vi "Handle.vi"(10 "log record":T1 {"timestamp" format="%<%x %.3X>T"}, 11 "logger in":refnum<class "Logger.lvclass">) -> (3 "logger out":refnum<class "Logger.lvclass">)   [LabVIEW 2024, in "Logging.lvlib" / "Logger.lvclass"]
uses:
  Logger.lvclass
  Log Record.ctl
  Internal Log Levels.ctl
  Logger.lvclass/Logger.ctl
  Failure Popup.vi
  <vilib>/ErrorRing/Error Ring.xnode
  Handlers/Handler/Handler.lvclass
  Logging.lvlib
panel:
  # "Connector Pane"
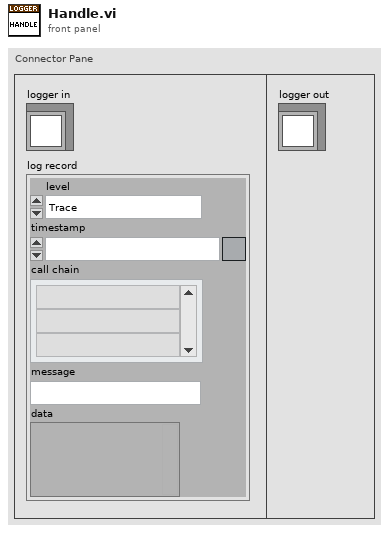
[diagram p1: front panel]
types:
  T1 = typedef "Logging.lvlib/Log Record.ctl" = cluster{"level":T2, "timestamp":timestamp, "call chain":string[], "message":string, "data":variant}
  T2 = typedef "Logging.lvlib/Internal Log Levels.ctl" = enum16{"Trace", "Debug", "Info", "Warning", "Error", "Critical", "Internal"}
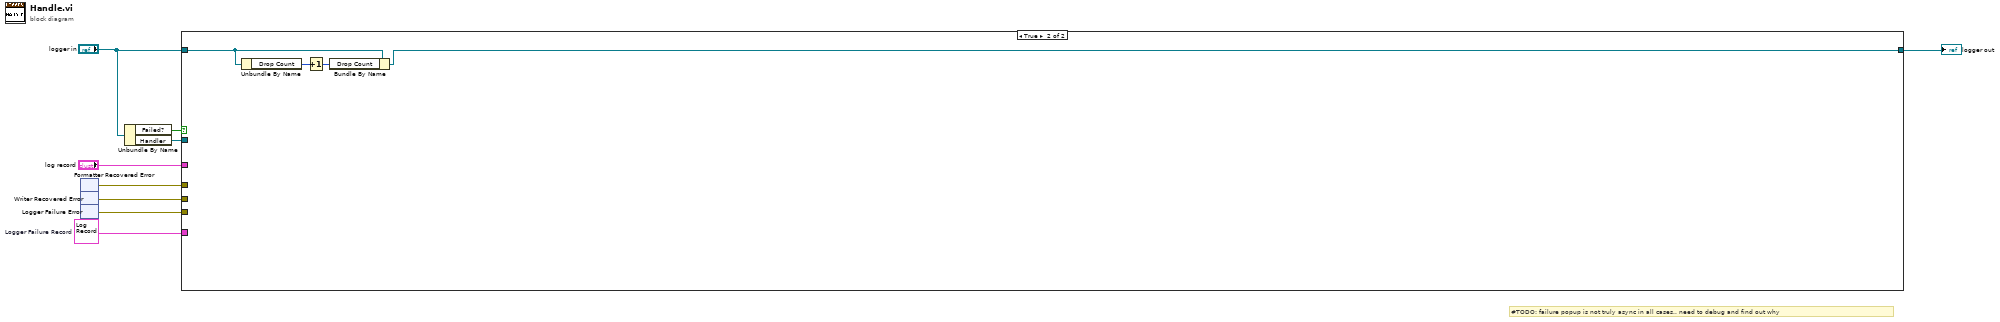
[diagram p0: block diagram]
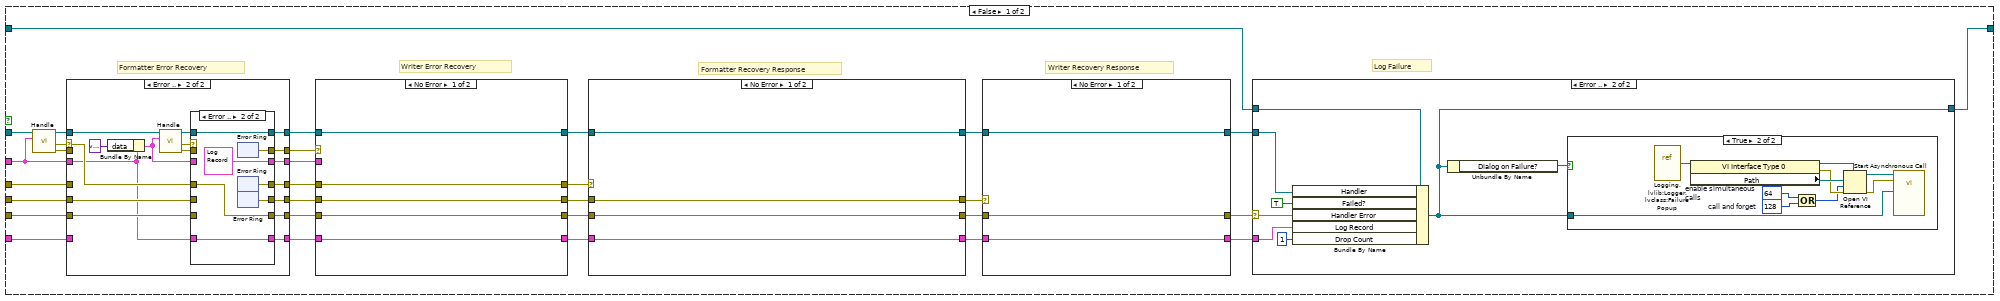
[diagram p2: hidden frame]
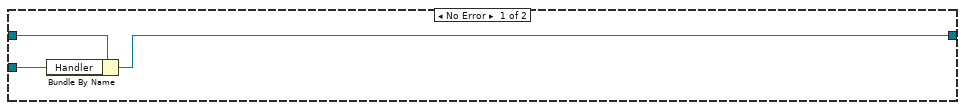
[diagram p3: hidden frame]
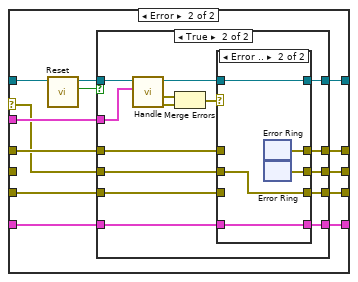
[diagram p7: hidden frame]
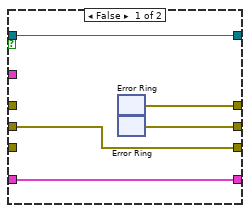
[diagram p8: hidden frame]
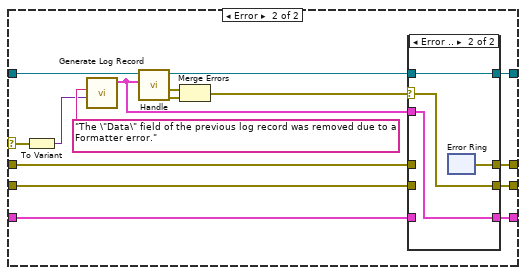
[diagram p10: hidden frame]
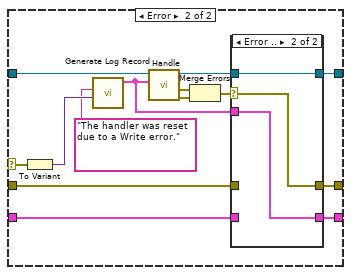
[diagram p12: hidden frame]
diagram:
  w9 = T1 {"level"=enum."Trace", "timestamp"=timestamp(0 s since 1904-01-01), "call chain"=[], "message"="", "data"=variant}  # Logger Failure Record
  # "#TODO: failure popup is not truly async in all cases.. need to debug and find out why"
  n1 = xnode "Formatter Recovered Error"() -> ("error out"=w6:errorcluster)
  n2 = xnode "Writer Recovered Error"() -> ("error out"=w7:errorcluster)
  n3 = xnode "Logger Failure Error"() -> ("error out"=w8:errorcluster)
  n4 = Unbundle By Name("logger in") -> ("Failed?"=w1:bool, "Handler"=w5:refnum<class "Handler.lvclass">)
  n5 = case shown="True" w1 {
    tunnel: w9 -> [w38 _]
    tunnel: w8 -> [w33 _]
    tunnel: w7 -> [w32 _]
    tunnel: w6 -> [w30 _]
    tunnel: w5 -> [w15 _]
    tunnel: "log record" -> [w13 _]
    tunnel: "logger in" -> [w11 w205]
    tunnel: [w10 w204] -> w2
    frame False {
      # "Log Failure"
      # "Writer Recovery Response"
      # "Formatter Recovery Response"
      # "Writer Error Recovery"
      # "Formatter Error Recovery"
      n6 = call-dynamic "Handle.vi"("log record"=w13, "handler in"=w15) -> ("writer error"=w16:errorcluster, "formatter error"=w12:errorcluster, "handler out"=w14:refnum<class "Handler.lvclass">)  [unwired: 7 in]
      n7 = case shown="Error .." w12 {
        selector: w12 -> [_ w69]
        tunnel: w13 -> [w61 w67]
        tunnel: w14 -> [w62 w82]
        tunnel: w16 -> [w66 _]
        tunnel: [w66 w79] -> w17
        tunnel: [w65 w78] -> w18
        tunnel: [w63 w76] -> w19
        tunnel: w30 -> [w65 _]
        tunnel: w33 -> [w63 w77]
        tunnel: [w64 w75] -> w24
        tunnel: w32 -> [w64 w74]
        tunnel: [w62 w73] -> w27
        tunnel: [w61 w70] -> w28
        tunnel: [w61 w68] -> w37
        tunnel: w38 -> [_ _]
        frame No Error {
        }
        frame Error {
          n8 = Bundle By Name(cluster=w67, "data"=variant) -> (w71:T1)
          n9 = call-dynamic "Handle.vi"("log record"=w71, "handler in"=w82) -> ("writer error"=w80:errorcluster, "formatter error"=w81:errorcluster, "handler out"=w72:refnum<class "Handler.lvclass">)  [unwired: 7 in]
          n10 = case shown="Error .." w81 {
            tunnel: w80 -> [w89 _]
            tunnel: [w89 w96] -> w79
            tunnel: [w85 w93] -> w78
            tunnel: [w88 w91] -> w76
            tunnel: w69 -> [w85 w91]
            tunnel: w77 -> [w88 _]
            tunnel: [w87 w92] -> w75
            tunnel: w74 -> [w87 _]
            tunnel: [w86 w95] -> w73
            tunnel: w72 -> [w86 w95]
            tunnel: [w84 T1 {"level"=enum."Trace", "timestamp"=timestamp(0 s since 1904-01-01), "call chain"=[], "message"="", "data"=variant} ("log record")] -> w70
            tunnel: w71 -> [w84 _]
            tunnel: [w84 w90] -> w68
            tunnel: w67 -> [_ w90]
            frame No Error {
            }
            frame Error {
              n11 = xnode "Error Ring"() -> ("error out"=w96:errorcluster)
              n12 = xnode "Error Ring"() -> ("error out"=w93:errorcluster)
              n13 = xnode "Error Ring"() -> ("error out"=w92:errorcluster)
            }
          }
        }
      }
      n14 = case shown="No Error" w17 {
        selector: w17 -> [_ w107]
        tunnel: w18 -> [w104 w112]
        tunnel: w19 -> [w103 w110]
        tunnel: [w104 w113] -> w20
        tunnel: [w103 w108] -> w23
        tunnel: [w102 w111] -> w26
        tunnel: w24 -> [w102 _]
        tunnel: w27 -> [w101 w117]
        tunnel: w28 -> [_ w114]
        tunnel: [w101 w109] -> w29
        tunnel: [w100 w106] -> w36
        tunnel: w37 -> [w100 w105]
        frame No Error {
        }
        frame Error {
          n15 = call-dynamic "Reset.vi"("handler in"=w117) -> ("successful?"=w115:bool, "handler out"=w116:refnum<class "Handler.lvclass">)  [unwired: 9 in]
          n16 = case shown="True" w115 {
            tunnel: w116 -> [w122 w139]
            tunnel: w114 -> [_ w135]
            tunnel: [w121 w134] -> w113
            tunnel: w112 -> [_ w133]
            tunnel: [w120 w132] -> w111
            tunnel: w107 -> [w119 w131]
            tunnel: w110 -> [_ w130]
            tunnel: [w122 w129] -> w109
            tunnel: [w119 w127] -> w108
            tunnel: [w118 w126] -> w106
            tunnel: w105 -> [w118 w125]
            frame False {
              n17 = xnode "Error Ring"() -> ("error out"=w121:errorcluster)
              n18 = xnode "Error Ring"() -> ("error out"=w120:errorcluster)
            }
            frame True {
              n19 = call-dynamic "Handle.vi"("log record"=w135, "handler in"=w139) -> ("writer error"=w137:errorcluster, "formatter error"=w138:errorcluster, "handler out"=w128:refnum<class "Handler.lvclass">)  [unwired: 7 in]
              n20 = Merge Errors(w138, w137) -> (w136:errorcluster)
              n21 = case shown="Error .." w136 {
                tunnel: [w144 w148] -> w134
                tunnel: w133 -> [w144 _]
                tunnel: [w141 w147] -> w132
                tunnel: w131 -> [w141 w146]
                tunnel: w130 -> [w142 _]
                tunnel: [w143 w149] -> w129
                tunnel: w128 -> [w143 w149]
                tunnel: [w142 w146] -> w127
                tunnel: [w140 w145] -> w126
                tunnel: w125 -> [w140 w145]
                frame No Error {
                }
                frame Error {
                  n22 = xnode "Error Ring"() -> ("error out"=w148:errorcluster)
                  n23 = xnode "Error Ring"() -> ("error out"=w147:errorcluster)
                }
              }
            }
          }
        }
      }
      n24 = case shown="No Error" w20 {
        selector: w20 -> [_ w170]
        tunnel: [w155 w159] -> w22
        tunnel: w23 -> [w155 w163]
        tunnel: [w154 w160] -> w25
        tunnel: w26 -> [w154 w168]
        tunnel: w29 -> [w153 w171]
        tunnel: [w153 w161] -> w31
        tunnel: [w152 w158] -> w35
        tunnel: w36 -> [w152 w157]
        frame No Error {
        }
        frame Error {
          n25 = To Variant(anything=w170) -> (Variant=w162:variant)
          n26 = call "Generate Log Record.vi"("data (null)"=w162, "message (\"\")"="The \"Data\" field of the previous log record was removed due to a Formatter error." ("message (\"\")")) -> ("log record"=w156:T1)  [unwired: 9 in]
          n27 = call-dynamic "Handle.vi"("log record"=w156, "handler in"=w171) -> ("writer error"=w166:errorcluster, "formatter error"=w167:errorcluster, "handler out"=w164:refnum<class "Handler.lvclass">)  [unwired: 7 in]
          n28 = Merge Errors(w167, w166) -> (w165:errorcluster)
          n29 = case shown="Error .." w165 {
            selector: w165 -> [_ w177]
            tunnel: w168 -> [w174 _]
            tunnel: w164 -> [w175 w179]
            tunnel: w163 -> [w173 _]
            tunnel: [w175 w179] -> w161
            tunnel: [w174 w178] -> w160
            tunnel: [w173 w177] -> w159
            tunnel: [w172 w176] -> w158
            tunnel: w157 -> [w172 _]
            tunnel: w156 -> [_ w176]
            frame No Error {
            }
            frame Error {
              n30 = xnode "Error Ring"() -> ("error out"=w178:errorcluster)
            }
          }
        }
      }
      n31 = case shown="No Error" w25 {
        selector: w25 -> [_ w191]
        tunnel: [w183 w188] -> w21
        tunnel: w22 -> [w183 w190]
        tunnel: w31 -> [w181 w192]
        tunnel: [w182 w187] -> w34
        tunnel: w35 -> [w182 w186]
        tunnel: [w181 w184] -> w39
        frame No Error {
        }
        frame Error {
          n32 = To Variant(anything=w191) -> (Variant=w193:variant)
          n33 = call "Generate Log Record.vi"("data (null)"=w193, "message (\"\")"="The handler was reset due to a Write error." ("message (\"\")")) -> ("log record"=w185:T1)  [unwired: 9 in]
          n34 = call-dynamic "Handle.vi"("log record"=w185, "handler in"=w192) -> ("writer error"=w196:errorcluster, "formatter error"=w197:errorcluster, "handler out"=w194:refnum<class "Handler.lvclass">)  [unwired: 7 in]
          n35 = Merge Errors(w197, w196) -> (w195:errorcluster)
          n36 = case shown="Error .." w195 {
            selector: w195 -> [_ w202]
            tunnel: w194 -> [w200 w203]
            tunnel: w190 -> [w199 _]
            tunnel: [w200 w203] -> w184
            tunnel: [w199 w202] -> w188
            tunnel: [w198 w201] -> w187
            tunnel: w186 -> [w198 _]
            tunnel: w185 -> [_ w201]
            frame No Error {
            }
            frame Error {
            }
          }
        }
      }
      n37 = case shown="Error .." w21 {
        selector: w21 -> [_ w47]
        tunnel: w11 -> [w42 w50]
        tunnel: w34 -> [_ w48]
        tunnel: [w41 w44] -> w10
        tunnel: w39 -> [w40 w45]
        frame No Error {
          n38 = Bundle By Name(cluster=w42, "Handler"=w40) -> (w41:refnum<class "Logger.lvclass">)
        }
        frame Error {
          n39 = Bundle By Name(cluster=w50, "Handler"=w45, "Failed?"=TRUE, "Handler Error"=w47, "Log Record"=w48, "Drop Count"=u32 1 ("Fail Info.Drop Count")) -> (w44:refnum<class "Logger.lvclass">)
          n40 = Unbundle By Name(w44) -> ("Dialog on Failure?"=w43:bool)
          n41 = case shown="True" w43 {
            tunnel: w44 -> [_ w54]
            frame False {
            }
            frame True {
              w52 = 128  # call and forget
              w53 = 64  # enable simultaneous calls
              n42 = vi-ref "Logging.lvlib:Logger.lvclass:Failure Popup.vi"() -> (w60:refnum<vi>)
              n43 = property class="VI Interface Type 0"(reference=w60) -> (reference out=w57:refnum<vi>, error out=w58:errorcluster, "Path"=w59:path)  [unwired: 1 in]
              n44 = Compound Arithmetic op=OR(w53, w52) -> (w51:i32)
              n45 = Open VI Reference(type specifier VI Refnum (for type only)=w57, vi path=w59, options=w51, error in (no error)=w58) -> (vi reference=w55:refnum<vi>, error out=w56:errorcluster)  [unwired: 2 in]
              n46 = call-by-ref "Start Asynchronous Call"(reference=w55, error in=w56, "Logger in"=w54) -> ()  [unwired: 11 in, 2 out]
            }
          }
        }
      }
    }
    frame True {
      n47 = Unbundle By Name(w205) -> ("Drop Count"=w207:u32)
      n48 = Increment(x=w207) -> (x+1=w206:u32)
      n49 = Bundle By Name(cluster=w205, "Drop Count"=w206) -> (w204:refnum<class "Logger.lvclass">)
    }
  }
  "logger out" <- w2
